vi "RS485TestRx.vi"(8 "error in (no error)":errorcluster, 9 "value":string, 10 "method":string, 11 "Sequence Context In":refnum<k7>) -> (0 "error out":errorcluster, 2 "status":string, 3 "Description":string)   [LabVIEW 2021]
uses:
  <vilib>/addons/TestStand/_TSUtility.llb/TestStand - Get Property Value (String).vi
  <vilib>/NI/JSON Support for LabVIEW/JSON Value/New JSON Value/New JSON ({String}).vi
  <vilib>/NI/NI JSONRPC Server Framework/Classes/Client/Format Client Request (Auto-Increment).vi
  <vilib>/NI/JSON Support for LabVIEW/JSON Value/JSON Value.lvclass
  <vilib>/NI/NI JSONRPC Server Framework/Classes/Client/JSONRPC Client.lvclass
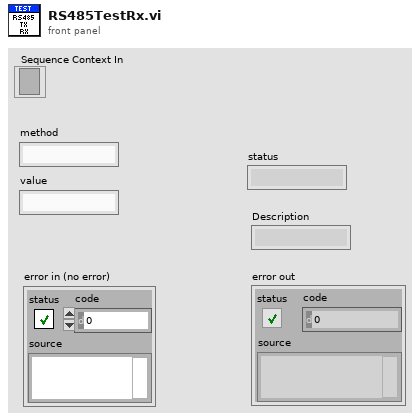
[diagram p1: front panel]
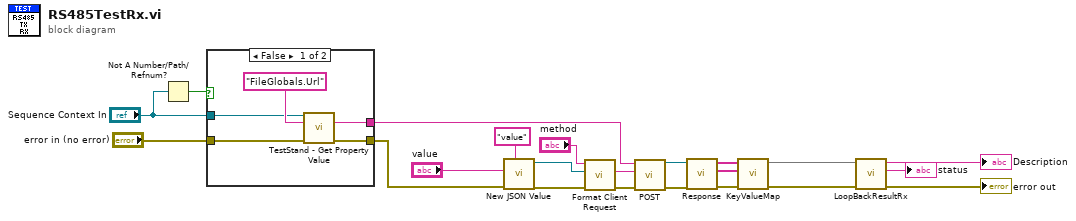
[diagram p0: block diagram]
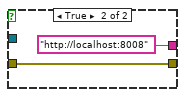
[diagram p2: hidden frame]
diagram:
  n1 = Not A Number/Path/Refnum?(number/path/refnum="Sequence Context In") -> (NaN/Path/Refnum?=w3:bool)
  n2 = case shown="False" w3 {
    tunnel: [w26 "http://localhost:8008" ("Value")] -> w22
    tunnel: [w25 w28] -> w21
    tunnel: "error in (no error)" -> [w24 w28]
    tunnel: "Sequence Context In" -> [w23 _]
    frame False {
      n3 = call-poly <vilib>:"TestStand - Get Property Value.vi"("Sequence Context In"=w23, "Lookup String"="FileGlobals.Url", "error in (no error)"=w24) -> ("Value"=w26:string, "error out"=w25:errorcluster)  [unwired: 10 in, 1 out]
    }
    frame True {
    }
  }
  n4 = call-poly <vilib>:"New JSON Value.vi"("key"="value", "error in (no error)"=w21, "value"="value") -> ("error out"=w9:errorcluster, "JSON Value out"=w8:refnum<class "JSON Value.lvclass">)  [unwired: 7 in]
  n5 = call-poly <vilib>:"Format Client Request.vi"("error in (no error)"=w9, "JSON Value in"=w8, "method"="method") -> ("error out"=w11:errorcluster, "Request String"=w12:string)  [unwired: 7 in]
  n6 = call "POST.vi"("error in (no error)"=w11, "Request String"=w12, "url"=w22) -> ("error out"=w13:errorcluster, "JSON Value out"=w14:refnum<class "JSON Value.lvclass">)  [unwired: 7 in]
  n7 = call "Response.vi"("error in (no error)"=w13, "JSON Value in"=w14) -> ("error out"=w15:errorcluster, "values"=w17:string[], "keys"=w16:string[])  [unwired: 7 in]
  n8 = call "KeyValueMap.vi"("error in"=w15, "values"=w17, "keys"=w16) -> ("error out"=w6:errorcluster, "map out"=w7:map{string, string})  [unwired: 7 in]
  n9 = call "LoopBackResultRx.vi"("error in (no error)"=w6, "map"=w7) -> ("error out"=→"error out":errorcluster, "status"=→"status":string, "description"=→"Description":string)  [unwired: 7 in]
